vi "AVI-AVI2 Open all.vi"(8 "error in (no error)":errorcluster, 11 "First AVI2 video's Path":path) -> (0 "error out":errorcluster, 1 "Number of frames in each AVI2 file":u32[](array[numeric]), 2 "Number of Frames (across all split videos)":u32, 3 "AVI2 split file refs":T1[](array[typedef]), 4 "Reinitialising in AVI1 mode":bool)   [LabVIEW 2013]
uses:
  <vilib>/vision/Avi.llb/IMAQ AVI2 Refnum.ctl
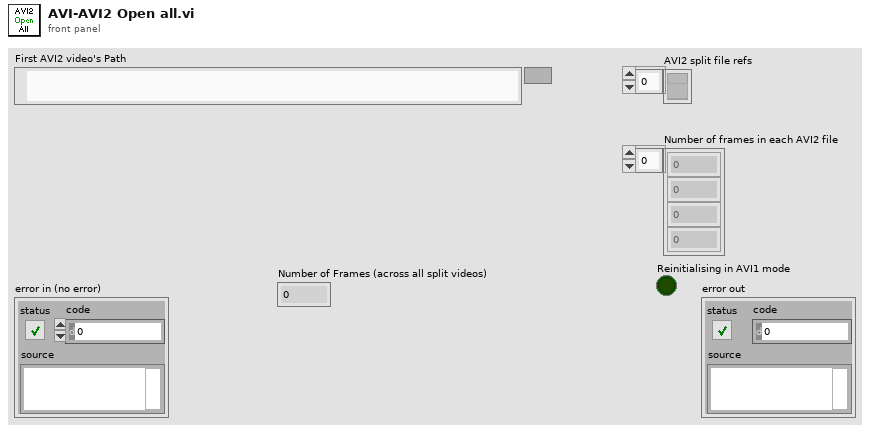
[diagram p1: front panel]
types:
  T1 = typedef "IMAQ AVI2 Refnum.ctl" = refnum<k20>
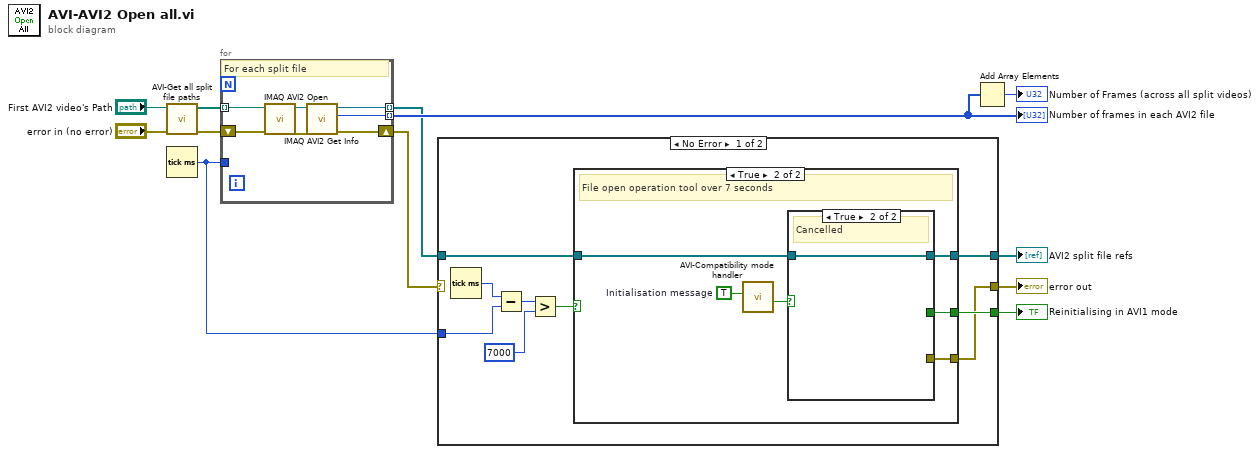
[diagram p0: block diagram]
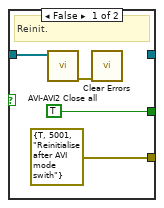
[diagram p3: hidden frame]
diagram:
  n1 = call "AVI-Get all split file paths.vi"("error in (no error)"="error in (no error)", "AVI2 video Path"="First AVI2 video's Path") -> ("error out"=w7:errorcluster, "Split AVI files path&name"=w9:path[])  [unwired: 8 in]
  n2 = Tick Count (ms)() -> (millisecond timer value=w6:u32)
  n3 = for {
    tunnel: [w16] -> w2 mode=indexing
    tunnel: w9 -> [w15] mode=indexing
    tunnel: [w14] -> w12 mode=indexing
    shift-right: [w17] -> w4
    shift-left: w7 -> [w13]
    tunnel: w6 -> [_]
    # "For each split file"
    n4 = call "IMAQ AVI2 Open"("error in (no error)"=w13, "AVI File Path"=w15) -> ("error out"=w18:errorcluster, "AVI Refnum"=w19:T1)  [unwired: 8 in]
    n5 = call "IMAQ AVI2 Get Info"("error in (no error)"=w18, "AVI Refnum"=w19) -> ("error out"=w17:errorcluster, "Number of Frames"=w14:u32, "AVI Refnum (duplicate)"=w16:T1)  [unwired: 5 in, 2 out]
  }
  "Number of frames in each AVI2 file" <- w12
  n6 = case shown="No Error" w4 {
    selector: w4 -> [_ w42]
    tunnel: w6 -> [w28 _]
    tunnel: [w27 _] -> w5
    tunnel: [w22 w42] -> w3
    tunnel: w2 -> [w21 w41]
    tunnel: [w20 w41] -> w1
    frame No Error {
      n7 = Tick Count (ms)() -> (millisecond timer value=w26:u32)
      n8 = Subtract(x=w26, y=w28) -> (x-y=w25:u32)
      n9 = Greater?(x=w25, y=u32 7000) -> (0:w23:bool)
      n10 = case shown="True" w23 {
        tunnel: [_ w33] -> w27
        tunnel: [_ w32] -> w22
        tunnel: w21 -> [w29 w31]
        tunnel: [w29 w30] -> w20
        frame False {
        }
        frame True {
          w35 = TRUE  # Initialisation message
          # "File open operation tool over 7 seconds"
          n11 = call "AVI-Compatibility mode handler.vi"("Initialisation message"=w35) -> ("Cancelled"=w34:bool)  [unwired: 10 in]
          n12 = case shown="True" w34 {
            tunnel: [TRUE _] -> w33
            tunnel: [errorcluster {"status"=TRUE, "code"=5001, "source"="Reinitialise after AVI mode swith"} ("error IO") _] -> w32
            tunnel: w31 -> [w37 w40]
            tunnel: [_ w40] -> w30
            frame False {
              # "Reinit."
              n13 = call "AVI-AVI2 Close all.vi"("AVI2 ref"=w37) -> ("error out"=w36:errorcluster)  [unwired: 10 in]
              n14 = call <vilib>:"Clear Errors.vi"("error in (no error)"=w36) -> ()  [unwired: 6 in, 1 out]
            }
            frame True {
              # "Cancelled"
            }
          }
        }
      }
    }
    frame Error {
    }
  }
  "AVI2 split file refs" <- w1
  "error out" <- w3
  "Reinitialising in AVI1 mode" <- w5
  n15 = Add Array Elements(numeric array=w12) -> (sum=→"Number of Frames (across all split videos)":u32)
